vi "getusercluster.vi"(10 "username":string, 11 "multiplayer":T1 {"player"."status" items=["host_ready", "idle", "host", "leaved", "ready", "playing", "lose(mine)", "lose(ot)", "win"]}) -> (3 "Numeric":i32)   [LabVIEW 2025]
uses:
  controls/playerstatus.ctl
  multi.ctl
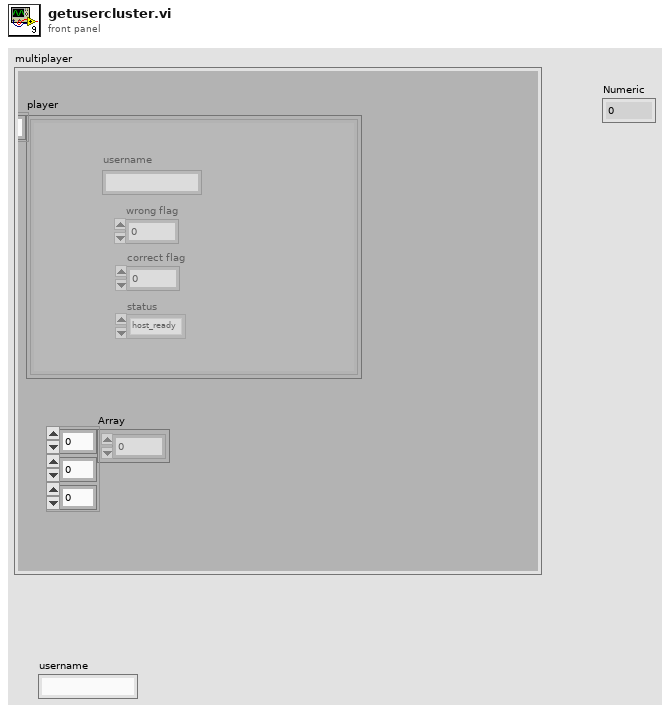
[diagram p1: front panel]
types:
  T1 = typedef "multi.ctl" = cluster{"Array":i8[][][], "player":T2[]}
  T2 = typedef "playerstatus.ctl" = cluster{"correct flag":i32, "wrong flag":i32, "username":string, "status":u16}
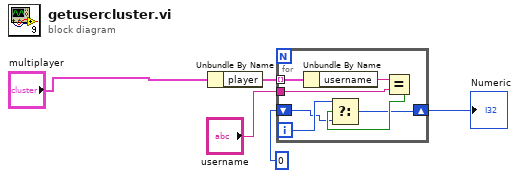
[diagram p0: block diagram]
diagram:
  n1 = Unbundle By Name("multiplayer") -> ("player"=w4:T2[])
  n2 = for {
    tunnel: w4 -> [w12] mode=indexing
    tunnel: "username" -> [w10]
    shift-right: [w6] -> w2
    shift-left: 0 -> [w7]
    i -> [w8]
    n3 = Unbundle By Name(w12) -> ("username"=w11:string)
    n4 = Equal?(x=w11, y=w10) -> (x = y?=w9:bool)
    n5 = Select(t=w8, s=w9, f=w7) -> (s? t:f=w6:i32)
  }
  "Numeric" <- w2
